vi "正弦波.vi"() -> ()   [LabVIEW 2017]
panel:
  in  "布尔":bool
  out "波形图表":dbl(graph)
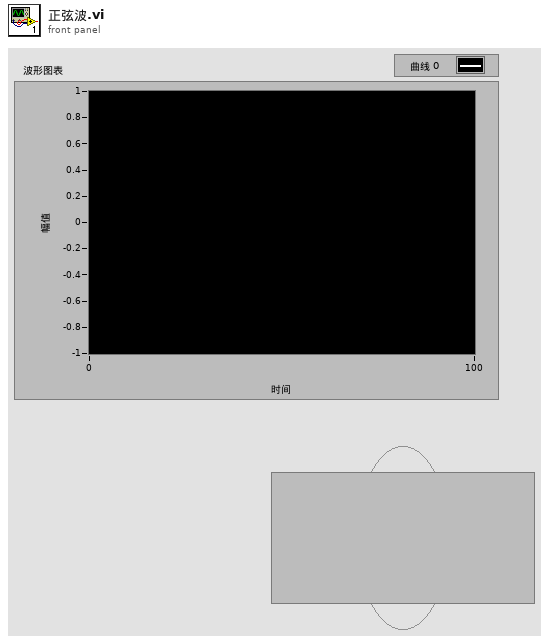
[diagram p1: front panel]
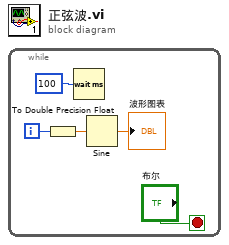
[diagram p0: block diagram]
diagram:
  n1 = while {
    i -> [w4]
    stop <- "布尔" stop-if-true
    n2 = To Double Precision Float(number=w4) -> (double precision float=w3:dbl)
    n3 = Wait (ms)(milliseconds to wait=u32 100 ("等待时间（毫秒）")) -> ()  [unwired: 1 out]
    n4 = Sine(x=w3) -> (sin(x)=→"波形图表":dbl)
  }
